vi "Write CSV File_2D.vi"(7 "delimiter (,)":string=",", 8 "error in (no error)":errorcluster, 9 "append to file? (new file)":bool, 10 "Array":dbl[][](array[numeric]), 11 "file path in":path) -> (0 "error out":errorcluster, 3 "file path out":path)   [LabVIEW 2017, in "Robust CSV.lvlib"]
doc: "Write a 2D array of strings to CSV file. The CSV file is formatted in accordance with RFC-4180 (see http://tools.ietf.org/html/rfc4180). \n\nA custom delimiter character can be specified. Default is a comma.\n\nSetting \"append to file?\" to true will append the data to the end of an existing file. Setting \"append to file?\" to false will overwrite an existing file. In both cases, if the file is not found, a new file will be created.\n\nRev 0.0 2014-02-20 Ryan Porter\n- First Draft\n\nRev 0.1 2014-10-30 Ryan Porter\n- Removed \"Convert EOL\" option from write to file to preserve compatibility with Excel CSV import."
uses:
  Robust CSV.lvlib
panel:
  # "Write CSV File_2D.vi\n\nWrite a 2D array of strings to CSV file. The CSV file is formatted in accordance with RFC-4180 (see http://tools.ietf.org/html/rfc4180). \n\nA custom delimiter character can be specified. Default is a comma.\n\nSetting \"append to file?\" to true will append the data to the end of an existing file. Setting \"append to file?\" to false will overwrite an existing file. In both cases, if the file is not found, a new file will be created."
  # "License: BSD (2-Clause) - http://opensource.org/licenses/BSD-2-Clause \n\nCopyright (c) 2014, Ryan Porter\nAll rights reserved."
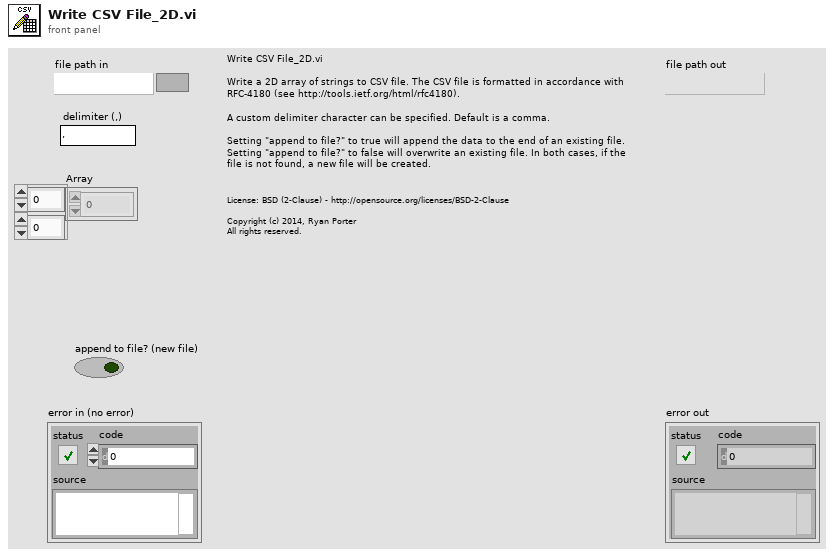
[diagram p1: front panel]
types:
  T1 = enum16{"open", "replace", "create", "open or create", "replace or create", "replace or create with confirmation"}
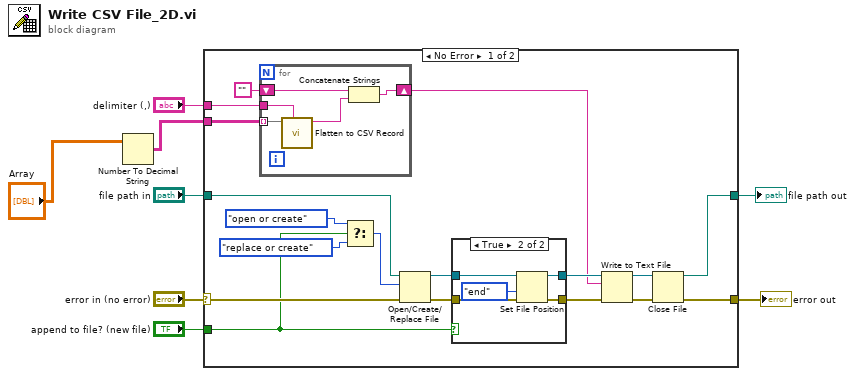
[diagram p0: block diagram]
diagram:
  n1 = Number To Decimal String(number="Array") -> (decimal integer string=w1:string[][])  [unwired: 1 in]
  n2 = case shown="No Error" "error in (no error)" {
    selector: "error in (no error)" -> [w24 w40]
    tunnel: "delimiter (,)" -> [w25 _]
    tunnel: [w13 w40] -> w6
    tunnel: "file path in" -> [w23 w39]
    tunnel: "append to file? (new file)" -> [w15 _]
    tunnel: [w10 w39] -> w3
    tunnel: w1 -> [w9 _]
    frame No Error {
      n3 = for {
        shift-right: [w37] -> w11
        shift-left: "" -> [w38]
        tunnel: w25 -> [w36]
        tunnel: w9 -> [w34] mode=indexing
        n4 = call "Flatten to CSV Record.vi"("delimiter (,)"=w36, "row of strings"=w34) -> ("CSV record"=w35:string)  [unwired: 8 in, 1 out]
        n5 = Concatenate Strings(w38, w35) -> (w37:string)
      }
      n6 = Select(t=T1."open or create" ("operation (0:open)"), s=w15, f=T1."replace or create" ("operation (0:open)")) -> (s? t:f=w20:T1)
      n7 = Open/Create/Replace File(file path (use dialog)=w23, error in=w24, operation (0:open)=w20) -> (refnum out=w19:refnum<file>, error out=w18:errorcluster)  [unwired: 3 in, 1 out]
      n8 = case shown="True" w15 {
        tunnel: w19 -> [w28 w33]
        tunnel: w18 -> [w27 w32]
        tunnel: [w27 w30] -> w17
        tunnel: [w28 w29] -> w16
        frame False {
        }
        frame True {
          n9 = Set File Position(refnum=w33, from (0:start)=enum16{"start", "end", "current"}."end", error in=w32) -> (refnum out=w29:refnum<file>, error out=w30:errorcluster)  [unwired: 1 in]
        }
      }
      n10 = Write to Text File(file (use dialog)=w16, text=w11, error in=w17) -> (refnum out=w12:refnum<file>, error out=w14:errorcluster)  [unwired: 1 in, 1 out]
      n11 = Close File(refnum=w12, error in=w14) -> (path=w10:path, error out=w13:errorcluster)
    }
    frame Error {
    }
  }
  "error out" <- w6
  "file path out" <- w3
